vi "Entanglement Table - Display.vi"(7 "QuWire in":refnum<class "QuWire.lvclass">) -> ()   [LabVIEW 2020]
uses:
  QuSim/QuWire/QuWire.lvclass
panel:
  out "Mutual Information":string[][](table)
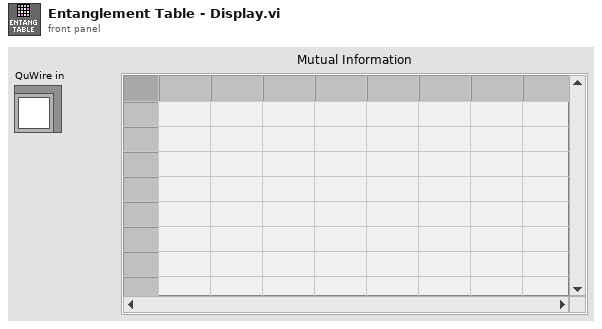
[diagram p1: front panel]
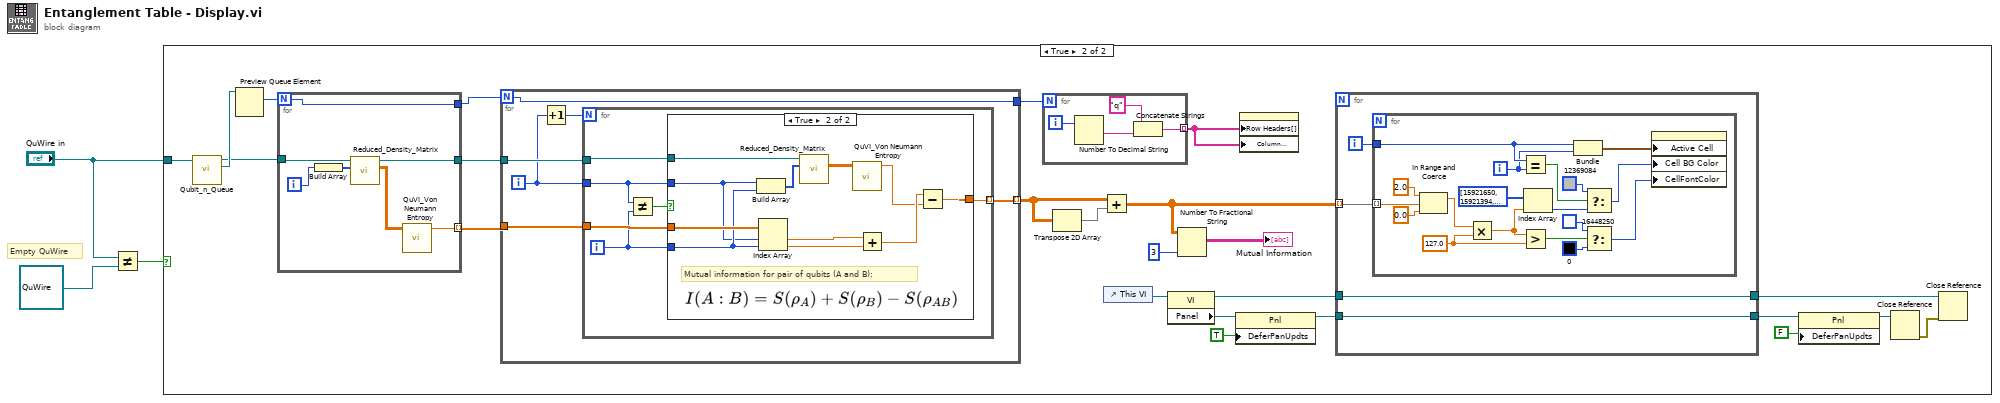
[diagram p0: block diagram]
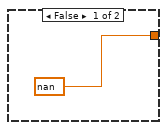
[diagram p3: hidden frame]
diagram:
  # "Empty QuWire"
  n1 = Not Equal?(x="QuWire in", y=refnum<class "QuWire.lvclass"> refnum ("QuWire in")) -> (x != y?=w1:bool)
  n2 = case shown="True" w1 {
    tunnel: "QuWire in" -> [_ w27]
    frame False {
    }
    frame True {
      n3 = call "Qubit_n_Queue.vi"("QuWire in"=w27) -> ("Qubit n"=w26:refnum<queue>, "QuWire out"=w24:refnum<class "QuWire.lvclass">)  [unwired: 8 in, 1 out]
      n4 = Preview Queue Element(queue=w26) -> (element=w25:i32)  [unwired: 2 in, 3 out]
      n5 = for {
        N: w25 -> [w30]
        tunnel: w24 -> [w32]
        tunnel: [w31] -> w23
        tunnel: [w30] -> w22
        tunnel: [w28] -> w21 mode=indexing
        i -> [w34]
        n6 = Build Array(w34) -> (w33:i32[])
        n7 = call "Reduced_Density_Matrix.vi"("Qubits to Keep"=w33, "QuWire in"=w32) -> ("Reduced Density Matrix"=w29:cdb[][], "QuWire out"=w31:refnum<class "QuWire.lvclass">)  [unwired: 6 in, 2 out]
        n8 = call "QuVI_Von Neumann Entropy.vi"("Density matrix"=w29) -> ("Von Neumann entropy"=w28:dbl)  [unwired: 10 in]
      }
      n9 = for {
        N: w22 -> [w39]
        tunnel: w23 -> [w44]
        tunnel: w21 -> [w43]
        tunnel: [w42] -> w19 mode=indexing
        tunnel: [w39] -> w4
        i -> [w41]
        n10 = Increment(x=w41) -> (x+1=w40:i32)
        n11 = for {
          N: w40 -> [_]
          tunnel: w44 -> [w50]
          tunnel: w43 -> [w49]
          tunnel: [w48] -> w42 mode=indexing
          tunnel: w41 -> [w45]
          i -> [w46]
          n12 = Not Equal?(x=w45, y=w46) -> (x != y?=w47:bool)
          n13 = case shown="True" w47 {
            tunnel: w50 -> [_ w61]
            tunnel: w49 -> [_ w59]
            tunnel: [nan w54] -> w48
            tunnel: w46 -> [_ w53]
            tunnel: w45 -> [_ w52]
            frame False {
            }
            frame True {
              # "Mutual information for pair of qubits (A and B):"
              n14 = Build Array(w52, w53) -> (w62:i32[])
              n15 = Index Array(array=w59, index #1=w52, index #2=w53) -> (element #1=w58:dbl, element #2=w57:dbl)
              n16 = call "Reduced_Density_Matrix.vi"("Qubits to Keep"=w62, "QuWire in"=w61) -> ("Reduced Density Matrix"=w60:cdb[][])  [unwired: 6 in, 3 out]
              n17 = call "QuVI_Von Neumann Entropy.vi"("Density matrix"=w60) -> ("Von Neumann entropy"=w55:dbl)  [unwired: 10 in]
              n18 = Add(x=w58, y=w57) -> (x+y=w56:dbl)
              n19 = Subtract(x=w56, y=w55) -> (x-y=w54:dbl)
            }
          }
        }
      }
      n20 = for {
        N: w4 -> [_]
        tunnel: [w37] -> w17 mode=indexing
        i -> [w38]
        n21 = Number To Decimal String(number=w38) -> (decimal integer string=w36:string)  [unwired: 1 in]
        n22 = Concatenate Strings("q" ("string"), w36) -> (w37:string)
      }
      n23 = Transpose 2D Array(2D array=w19) -> (transposed array=w20:dbl[][])
      n24 = Add(x=w19, y=w20) -> (x+y=w16:dbl[][])
      n25 = control-ref of="This VI"() -> (w15:refnum<vi>)
      n26 = property class="VI"(reference=w15) -> (reference out=w8:refnum<vi>, "Panel"=w14:refnum<vi>)  [unwired: 1 in, 1 out]
      n27 = Number To Fractional String(number=w16, precision (6)=i16 3) -> (F-format string=→"Mutual Information":string[][])  [unwired: 2 in]
      n28 = property class="Pnl"(reference=w14, "DeferPanUpdts"=TRUE ("Defer Panel Updates")) -> (reference out=w12:refnum<vi>)  [unwired: 1 in, 1 out]
      n29 = property on="Mutual Information" class="Tbl (strict)"("Row Headers[]"=w17, "Column Headers[]"=w17) -> ()  [unwired: 2 in, 2 out]
      n30 = for {
        tunnel: w16 -> [w66] mode=indexing
        tunnel: w12 -> [w64]
        tunnel: [w64] -> w11
        tunnel: w8 -> [w63]
        tunnel: [w63] -> w6
        i -> [w65]
        n31 = for {
          tunnel: w66 -> [w70] mode=indexing
          tunnel: w65 -> [w76]
          i -> [w75]
          w68 = 127.0 ("y")
          n32 = In Range and Coerce(upper limit=2.0, x=w70, lower limit=0.0) -> (coerced(x)=w69:dbl)  [unwired: 1 out]
          n33 = Multiply(x=w69, y=w68) -> (x*y=w67:dbl)
          n34 = Equal?(x=w76, y=w75) -> (x = y?=w74:bool)
          n35 = Greater?(x=w67, y=w68) -> (0:w83:bool)
          n36 = Index Array(array=u32[] [15921650, 15921394, 15921138, 15920882, 15920626, 15920370, 15854577, 15854065, 15853809, 15853553, 15853297, 15853041, 15852785, 15852529, 15852017, 15851761, 15851505, 15785712, 15785456, 15785200, 15784944, 15784688, 15784176, 15783920, 15783664, 15783408, 15783152, 15782896, 15782640, 15716847, 15716335, 15716335, 15715823, 15715567, 15715311, 15715055, 15714799, 15714543, 15714287, 15714031, 15647982, 15647726, 15647470, 15647214, 15646958, 15646702, 15646446, 15645934, 15645678, 15645422, 15645166, 15644910, 15579117, 15578861, 15578349, 15578093, 15577837, 15577581, 15577325, 15577069, 15576813, 15576301, 15576045, 15510252, 15509996, 15509740, 15509484, 15509228, 15508972, 15508460, 15508204, 15507948, 15507692, 15507436, 15507180, 15441387, 15441131, 15440619, 15440619, 15440107, 15439851, 15439595, 15439339, 15439083, 15438827, 15438571, 15438315, 15372266, 15372010, 15371754, 15371498, 15371242, 15370986, 15305193, 15239400, 15173864, 15108071, 15042534, 14976742, 14910949, 14910948, 14779619, 14714083, 14713826, 14648034, 14582497, 14516704, 14451168, 14385375, 14319582, 14254045, 14253789, 14122716, 14056923, 14056667, 13991130, 13925337, 13859544, 13794008, 13728215, 13662422, 13596886, 13596629, 13465556, 13399764, 13399763, 13333970, 13268178, 13202641, 13136848, 13071055, 13005519, 12939726, 12874189, 12808397, 12742604, 12742604, 12676811, 12611018, 12545481, 12479689, 12414152, 12348359, 12282567, 12217030, 12151237, 12151236, 12085444, 12019651, 11954114, 11888322, 11822529, 11756992, 11691200, 11625663, 11559870, 11494078, 11494077, 11428284, 11362747, 11296955, 11231162, 11165625, 11099833, 11034040, 10968504, 10902711, 10836918, 10836917, 10771125, 10705588, 10639795, 10574259, 10508466, 10442673, 10377136, 10311344, 10245551, 10180014, 10179758, 10114221, 10048428, 9982636, 9917099, 9851306, 9785514, 9719977, 9654184, 9588647, 9522855, 9522598, 9457061, 9391269, 9325732, 9259940, 9194147, 9128610, 9062817, 8997281, 8931488, 8931231, 8865695, 8799902, 8734109, 8668573, 8602780, 8536987, 8471450, 8405658, 8340121, 8274328, 8274072, 8208535, 8142742, 8077206, 8011413, 7945620, 7880083, 7814291, 7748754, 7682961, 7617169, 7617168, 7551376, 7485583, 7420046, 7354253, 7288717, 7222924, 7157131, 7091595, 7025802, 6960009, 6960009, 6894216, 6828679, 6762886, 6697094, 6631557, 6565764, 6500228, 6434435, 6368642, 6303106, 6302849, 6237312, 6171519, 6105727, 6040190, 5974398, 5908605, 5843068, 5777276, 5711483, 5645946, 5645689] ("Color table"), index=w67) -> (element=w78:u32)
          n37 = Bundle(w76, w75) -> (w84:cluster{i32, i32})  [unwired: 1 in]
          n38 = Select(t=u32 12369084, s=w74, f=w78) -> (s? t:f=w77:u32)
          n39 = Select(t=u32 16448250, s=w83, f=u32 0) -> (s? t:f=w80:u32)
          n40 = property on="Mutual Information" class="Tbl (strict)"("Active Cell"=w84, "Cell BG Color"=w77, "CellFontColor"=w80) -> ()  [unwired: 2 in, 2 out]
        }
      }
      n41 = property class="Pnl"(reference=w11, "DeferPanUpdts"=FALSE ("Defer Panel Updates")) -> (reference out=w9:refnum<vi>)  [unwired: 1 in, 1 out]
      n42 = Close Reference(reference=w9) -> (error out=w7:errorcluster)  [unwired: 1 in]
      n43 = Close Reference(reference=w6, error in (no error)=w7) -> ()  [unwired: 1 out]
    }
  }
